vi "Configure Output Impedance.vi"(8 "error in (no error)":errorcluster, 9 "Impedance (0: 50 Ohms)":u16(ring) items=["50 Ohms", "High Impedance"], 10 "Channel (0: Channel 1)":T1 items=["Channel 1", "Channel 2"], 11 "VISA resource name":refnum<visa-resource-name>) -> (0 "error out":errorcluster, 3 "VISA resource name out":refnum<visa-resource-name>)   [LabVIEW 2009, in "Tektronix AFG 3000 Series.lvlib"]
doc: "Configures the output impedance for the function generator."
uses:
  Tektronix AFG 3000 Series.lvlib
  controls.llb/Channel.ctl
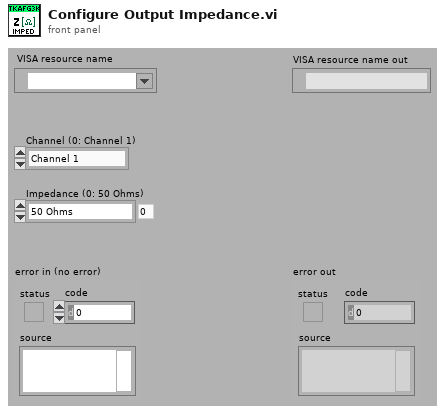
[diagram p1: front panel]
types:
  T1 = typedef "Channel.ctl" = u16
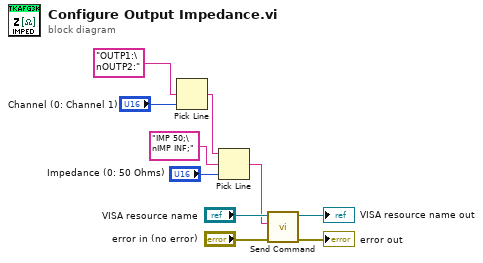
[diagram p0: block diagram]
diagram:
  n1 = Pick Line(multi-line string="OUTP1:\nOUTP2:" ("string (\"\")"), line index="Channel (0: Channel 1)") -> (output string=w6:string)  [unwired: 1 out]
  n2 = Pick Line(string ("")=w6, multi-line string="IMP 50;\nIMP INF;" ("Impedance Command"), line index="Impedance (0: 50 Ohms)") -> (output string=w3:string)
  n3 = call "Send Command.vi"("error in (no error)"="error in (no error)", "write buffer"=w3, "VISA resource name"="VISA resource name") -> ("error out"=→"error out":errorcluster, "VISA resource name out"=→"VISA resource name out":refnum<visa-resource-name>)  [unwired: 7 out]
